vi "Read Trial Config Info.vi"(11 "Test Trial File Name":string) -> (3 "Trial Settings OUT":T1={"Trial Label"="", "Type"="1.4", "Timeout (secs)"="", "Inter-Trial Interval (secs)"="", "Left Wall Enabled"=FALSE, "Right Wall Enabled"=FALSE, "Corridor Reset"=FALSE, "Default Wall Position"="", "Open Loop Change Positions"="", "Open Loop Values (mm)"="", "Corridor Width Change Positions"="", "Corridor Width Values (mm) "="", "Turn Change Positions"="0", "Turn Values (deg)"="1.4", "Left Texture Change Positions"="", "Right Texture Change Positions"="", "Video Frames (fps)"="", "Water Enabled"=FALSE, "Water Trial Position"="", "Photostimulation"="", "Water Corridor Max"="", "Water Range"="", "Water Drop Size (ms)"="", "Water Reward Position"="", "Duration (cm)"="", "Left Texture Enabled"=FALSE, "Right Texture Enabled"=FALSE, "Ps Trial Period"="", "Ps Inter-Pulse-Interval (ms)"="", "Ps Peak Power"="", "Ps Pulse Duration (ms)"="", "ephys_clock freq (hz)"="", "frame_clock (hz)"="", "Plot Color (Lateral Dist vs Trial Fraction)"=0})   [LabVIEW 2018]
uses:
  controls/Trial Config Settings.ctl
  controls/Command IN_Recipe.ctl
  Globals/Global - Configuration Options.vi
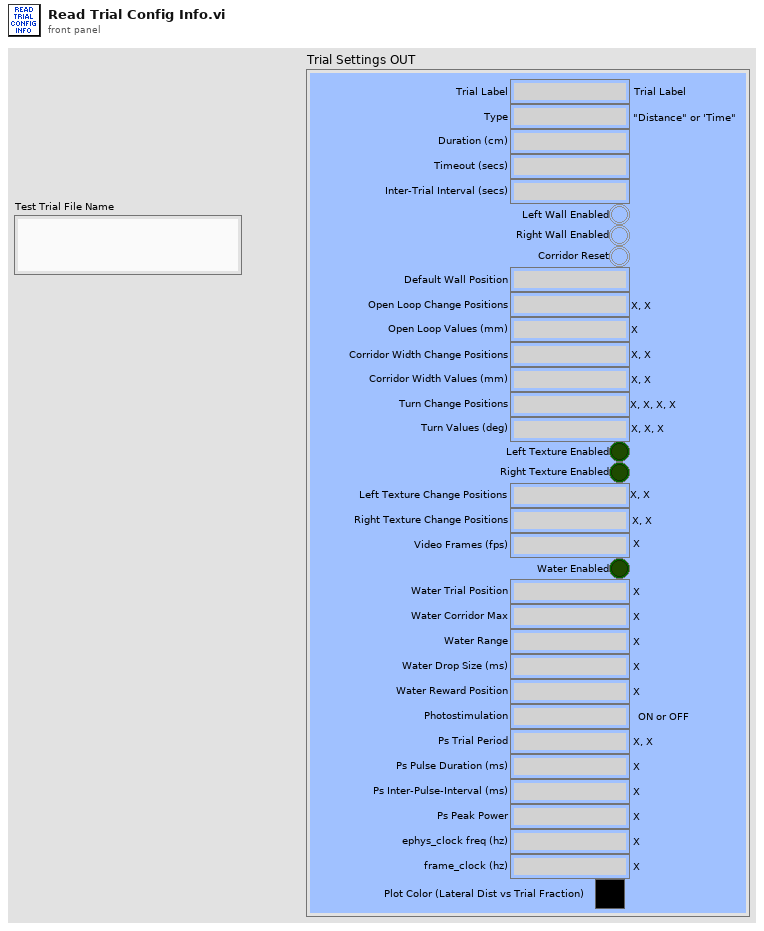
[diagram p1: front panel]
types:
  T1 = typedef "Trial Config Settings.ctl" = cluster{"Trial Label":string, "Type":string, "Timeout (secs)":string, "Inter-Trial Interval (secs)":string, "Left Wall Enabled":bool, "Right Wall Enabled":bool, "Corridor Reset":bool, "Default Wall Position":string, "Open Loop Change Positions":string, "Open Loop Values (mm)":string, "Corridor Width Change Positions":string, "Corridor Width Values (mm) ":string, "Turn Change Positions":string, "Turn Values (deg)":string, "Left Texture Change Positions":string, "Right Texture Change Positions":string, "Video Frames (fps)":string, "Water Enabled":bool, "Water Trial Position":string, "Photostimulation":string, "Water Corridor Max":string, "Water Range":string, "Water Drop Size (ms)":string, "Water Reward Position":string, "Duration (cm)":string, "Left Texture Enabled":bool, "Right Texture Enabled":bool, "Ps Trial Period":string, "Ps Inter-Pulse-Interval (ms)":string, "Ps Peak Power":string, "Ps Pulse Duration (ms)":string, "ephys_clock freq (hz)":string, "frame_clock (hz)":string, "Plot Color (Lateral Dist vs Trial Fraction)":u32}
  T2 = typedef "Command IN_Recipe.ctl" = enum16{"Save", "Load"}
  T3 = typedef "Rig Config Settings.ctl" = cluster{"Rig Name":string, "Rig Room":string, "Base Directory":string, "Computer IP Address":string, "Globals Name":string, "Treatmill Str":string, "cRIO Test Data Dir":path, "ai":string, "ao":string, "dio":string, "A_calib_str_row1":string, "A_calib_str_row2":string, "A_calib_str_row3":string, "Zero_V_str":string, "step_V":string, "Sample Freq":string, "ai_threshold":string, "run_speed_thresh":string, "speed_time_length":string, "wall ball gain":string, "max wall pos":string, "max cor width":string, "Trial Config Directory":path, "Randomize Trials?":bool}
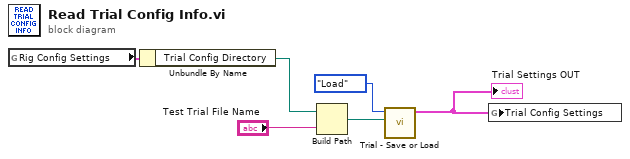
[diagram p0: block diagram]
diagram:
  n1 = global read "Global - Configuration Options.vi" "Rig Config Settings"() -> (w5:T3)
  n2 = Unbundle By Name(w5) -> ("Trial Config Directory"=w4:path)
  n3 = Build Path(base path=w4, name or relative path="Test Trial File Name") -> (appended path=w2:path)
  n4 = call "Trial - Save or Load.vi"("Trial Path IN"=w2, "Command IN"=Command_IN_Recipe."Load") -> ("Trial Settings OUT"=w1:T1)  [unwired: 8 in, 1 out]
  "Trial Settings OUT" <- w1
  n5 = global write "Global - Configuration Options.vi" "Trial Config Settings"(w1) -> ()
